vi "Dimostatore.vi"() -> ()   [LabVIEW 2019]
uses:
  ByteGSAPIBase/ByteGSAPIBase.lvclass
  ByteGSAPIBase/FetchCalibration/Converted_Slug_Cluster.ctl
  ByteGSAPIBase/CalibrationMeasurements/BodyCalibrazioneMisure.ctl
  6d3d0a70-a223-4ddd-b0d3-7207305fe689.vi
  85eea304-0067-4311-882a-d02f57de18c2.vi
panel:
  out "Valore misurato":string
  out "Valore di riferimento":string
  in  "Start":bool
  in  "Send":bool
  out "Infobox":string
  out "Strumenti da calibrare":i32(listbox)
  in  "Exit":bool=TRUE
  in  "Calibrate":bool
  in  "error out":errorcluster
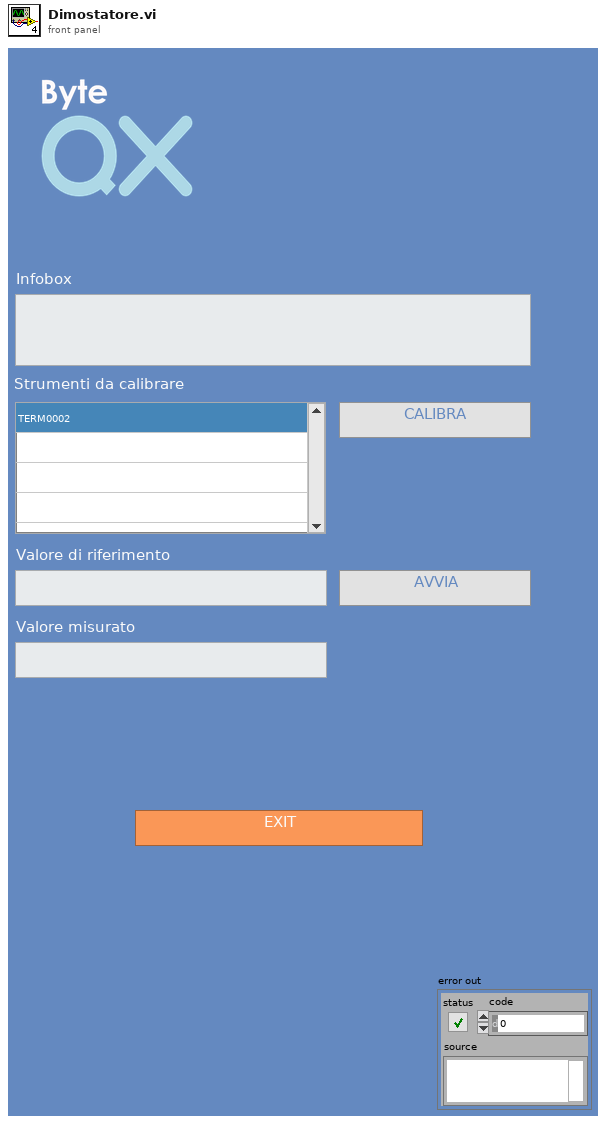
[diagram p1: front panel]
types:
  T1 = cluster{"nome":string, cluster{"Measurement_Id":i32, "Passed?":bool}[]}[]
  T2 = typedef "ByteGSWebAPI.lvlib/ByteGSAPIBase.lvclass/BodyCalibrazioneMisure.ctl" = cluster{"controls":cluster{"id":u16, "descrizione":string, "numero_misure_necessarie":u16, "riferimento_obiettivo":dbl, "mpe_max":dbl, "mpe_min":dbl, "deviazione_standard":dbl, "incertezza":dbl, "numero_misure_effettuate":u32, "temperatura_c":dbl, "umidita":dbl, "strumento_riferimento":cluster{"id":u16, "nome":string}[]}[]}
  T3 = typedef "ByteGSWebAPI.lvlib/ByteGSAPIBase.lvclass/Converted_Slug_Cluster.ctl" = cluster{"id":u32, "instrument":string, "name":string, "date":timestamp}
  T4 = cluster{"ByteGSAPIBase in":refnum<class "ByteGSAPIBase.lvclass">, "Expired_Instruments":T3[], "Calibrations":T2, "Strumenti_calibrati":cluster{"nome":string, cluster{"Measurement_Id":i32, "Passed?":bool}[]}[], "Instr_index":i32, "Calib_index":i32, "Instruments_Slug":string[], "ID_failed":u32, "Measure_Index":u32}
  T5 = cluster{"id":u16, "descrizione":string, "numero_misure_necessarie":u16, "riferimento_obiettivo":dbl, "mpe_max":dbl, "mpe_min":dbl, "deviazione_standard":dbl, "incertezza":dbl, "numero_misure_effettuate":u32, "temperatura_c":dbl, "umidita":dbl, "strumento_riferimento":cluster{"id":u16, "nome":string}[]}[]
  T6 = cluster{"id":u16, "descrizione":string, "numero_misure_necessarie":u16, "riferimento_obiettivo":dbl, "mpe_max":dbl, "mpe_min":dbl, "deviazione_standard":dbl, "incertezza":dbl, "numero_misure_effettuate":u32, "temperatura_c":dbl, "umidita":dbl, "strumento_riferimento":cluster{"id":u16, "nome":string}[]}
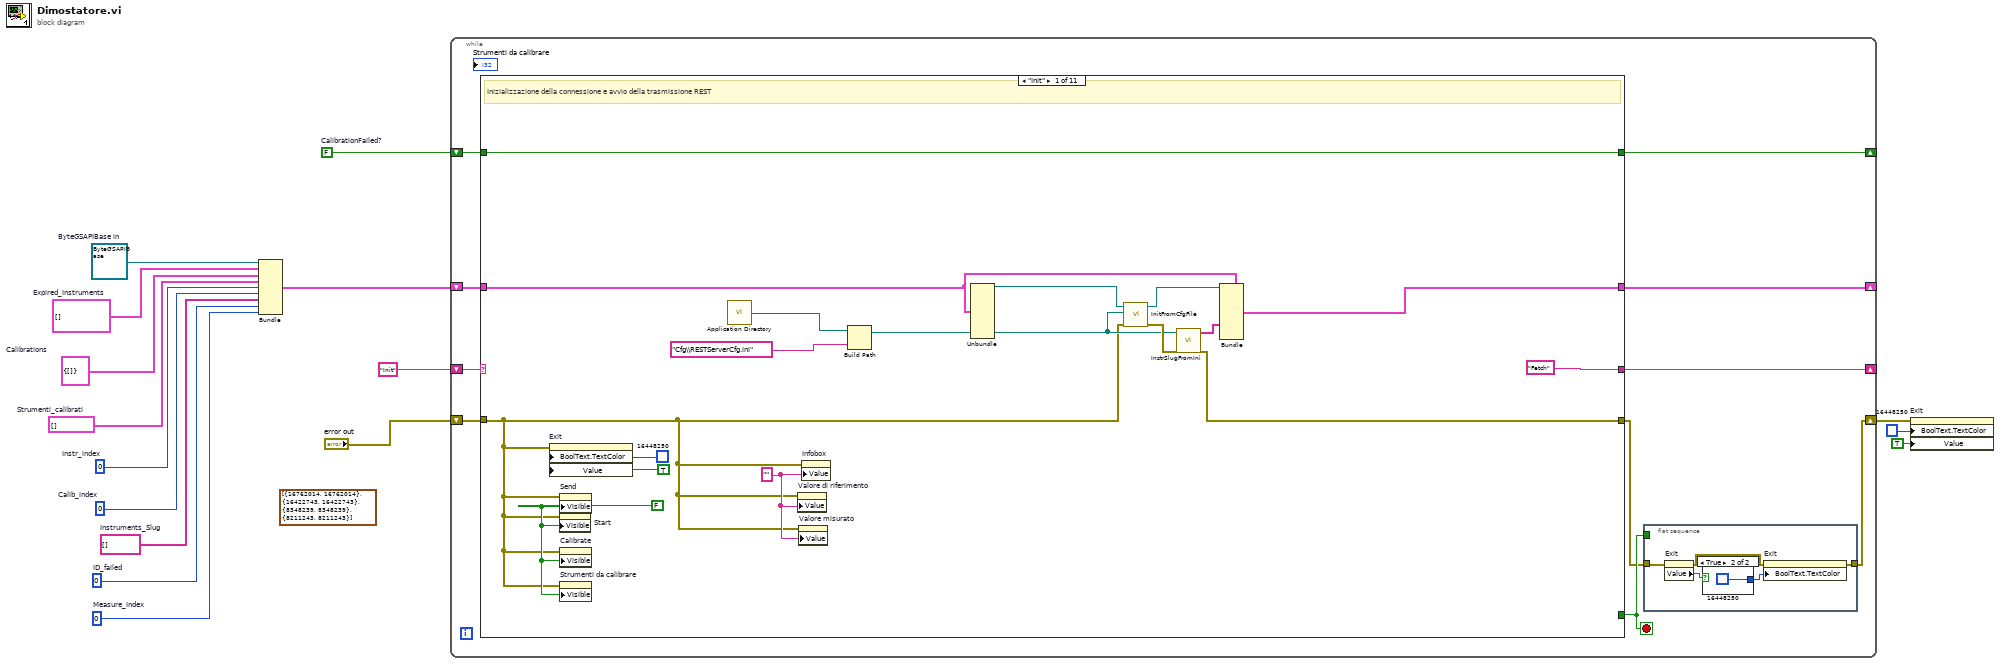
[diagram p0: block diagram]
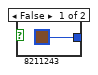
[diagram p2: hidden frame]
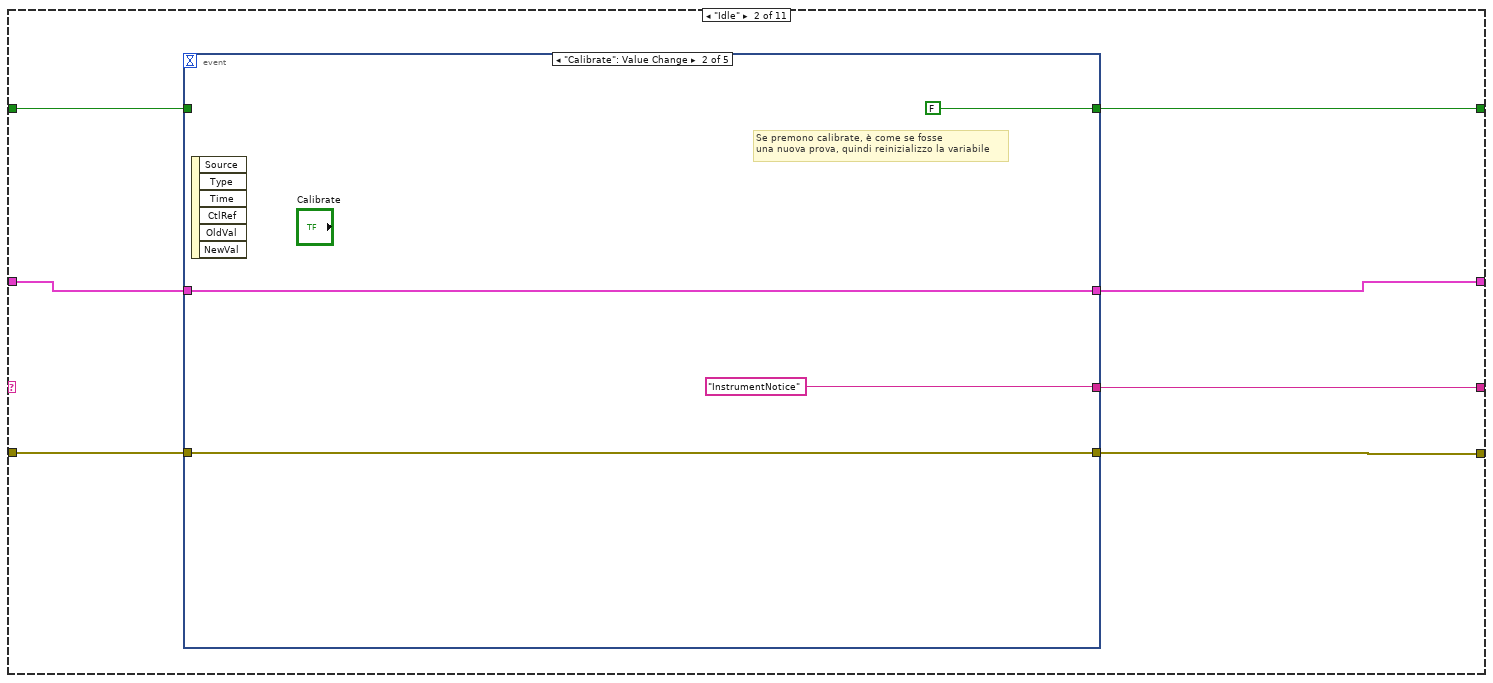
[diagram p3: hidden frame]
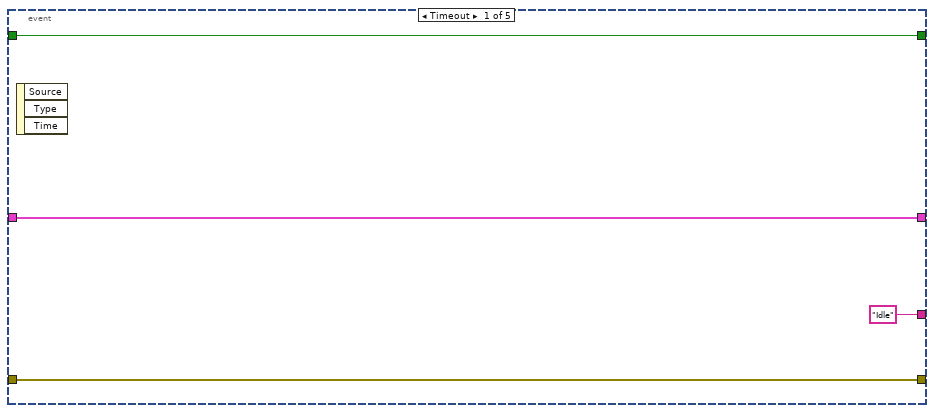
[diagram p4: hidden frame]
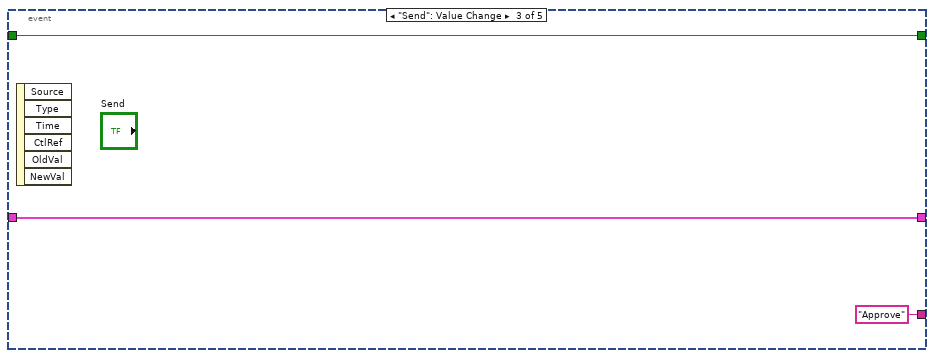
[diagram p5: hidden frame]
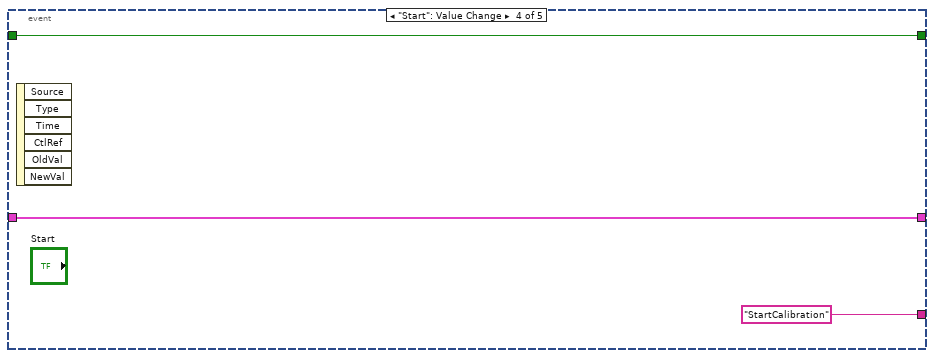
[diagram p6: hidden frame]
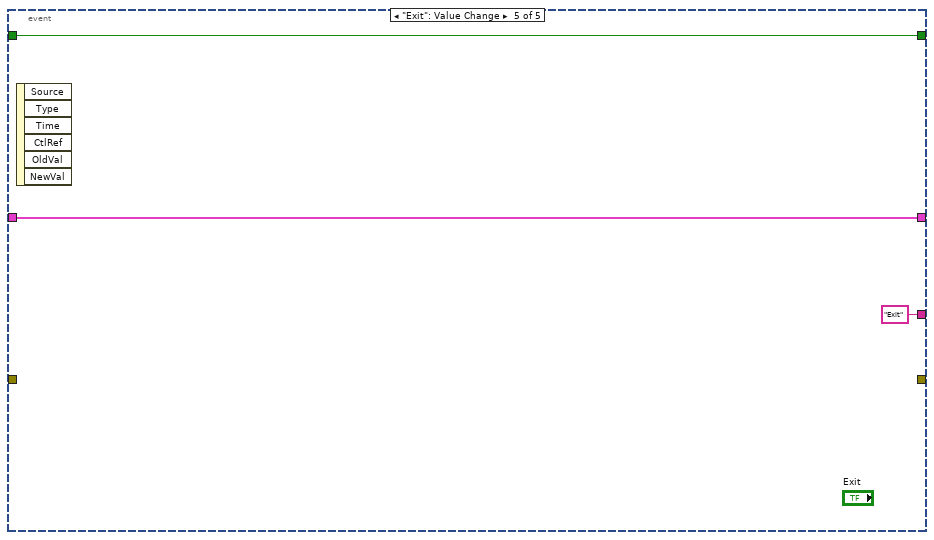
[diagram p7: hidden frame]
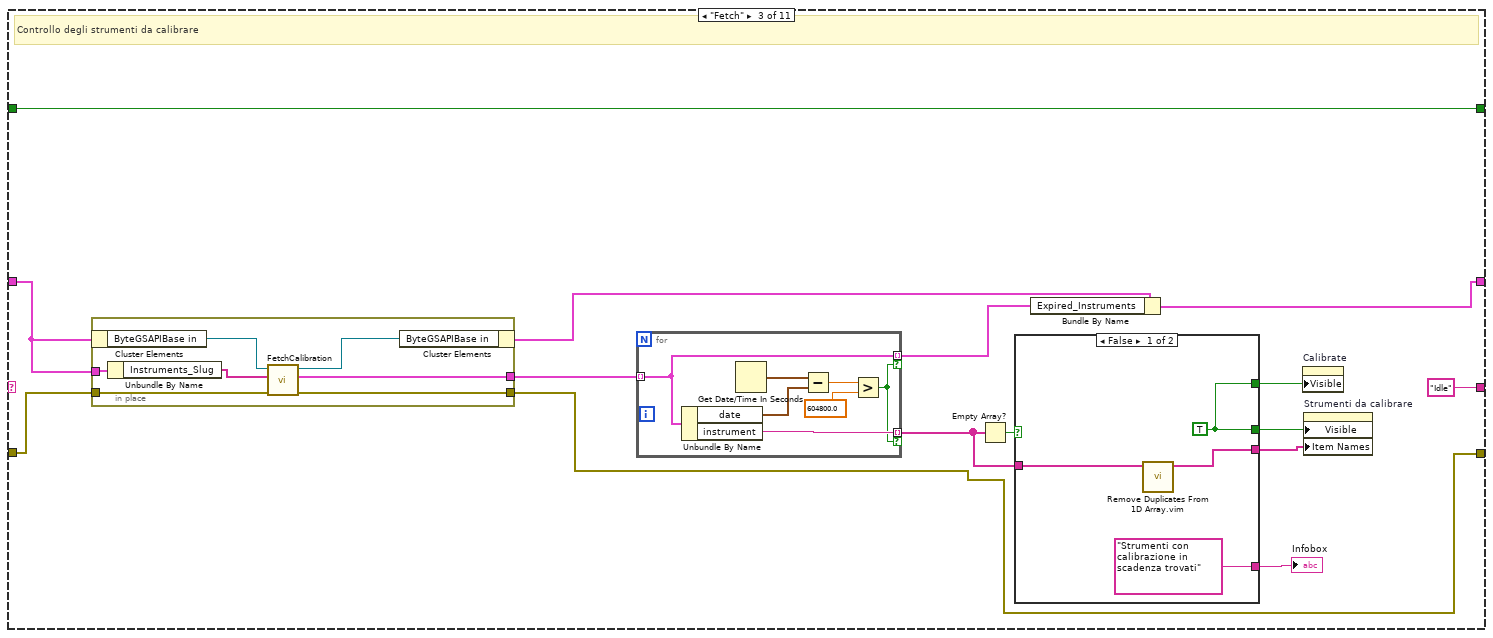
[diagram p8: hidden frame]
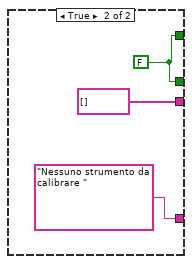
[diagram p9: hidden frame]
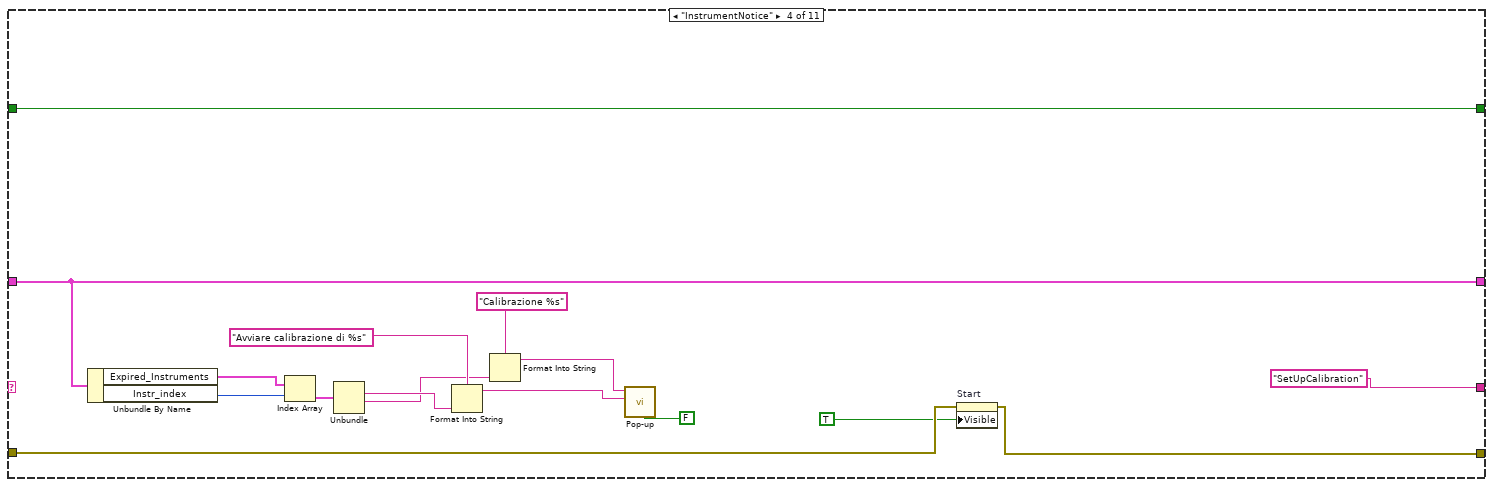
[diagram p10: hidden frame]
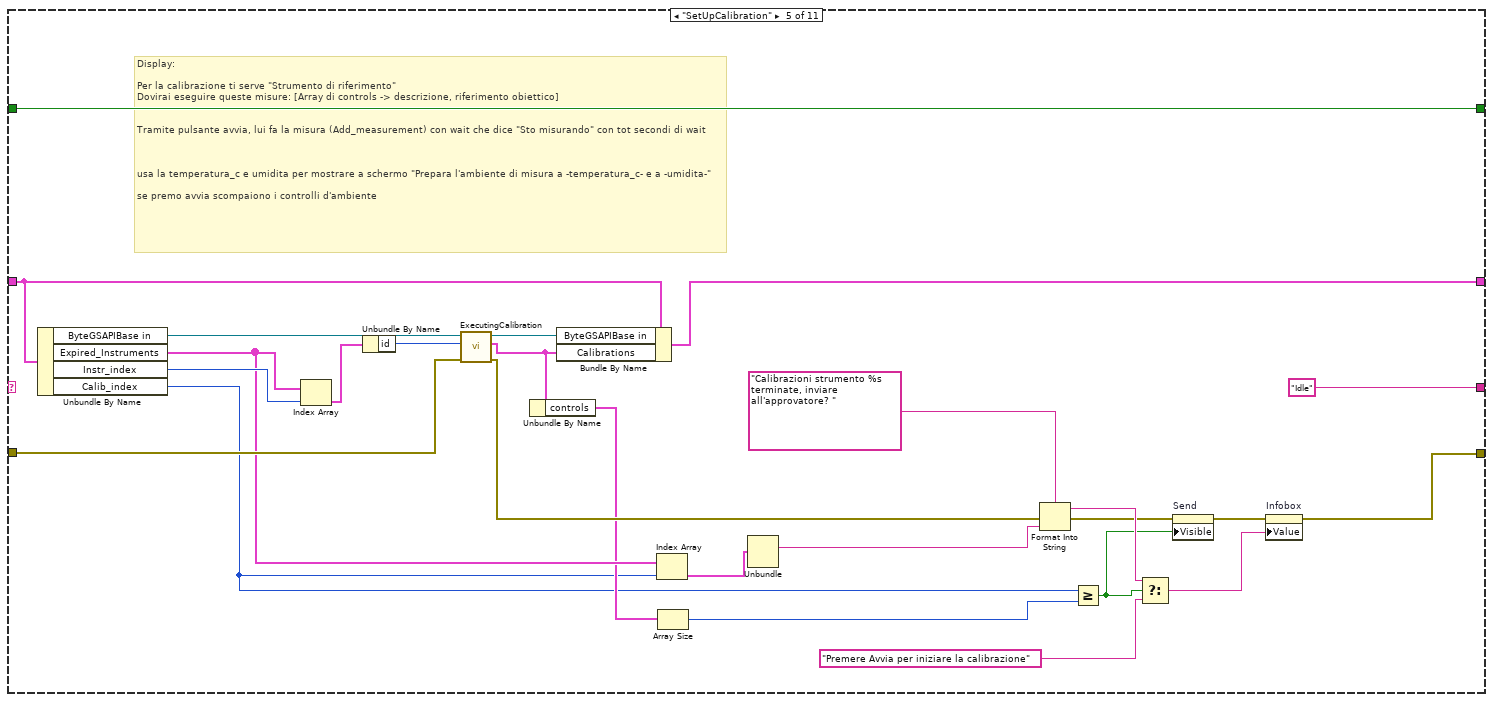
[diagram p11: hidden frame]
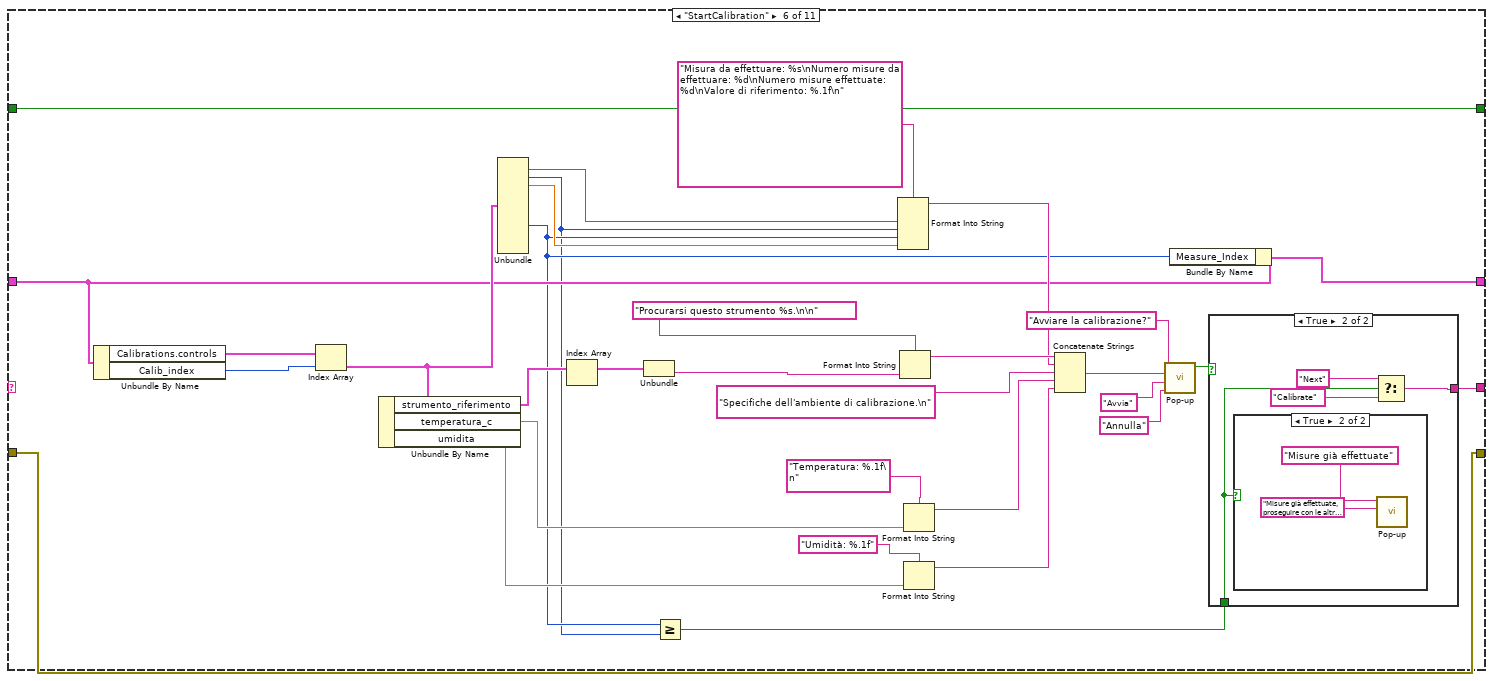
[diagram p12: hidden frame]
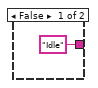
[diagram p13: hidden frame]
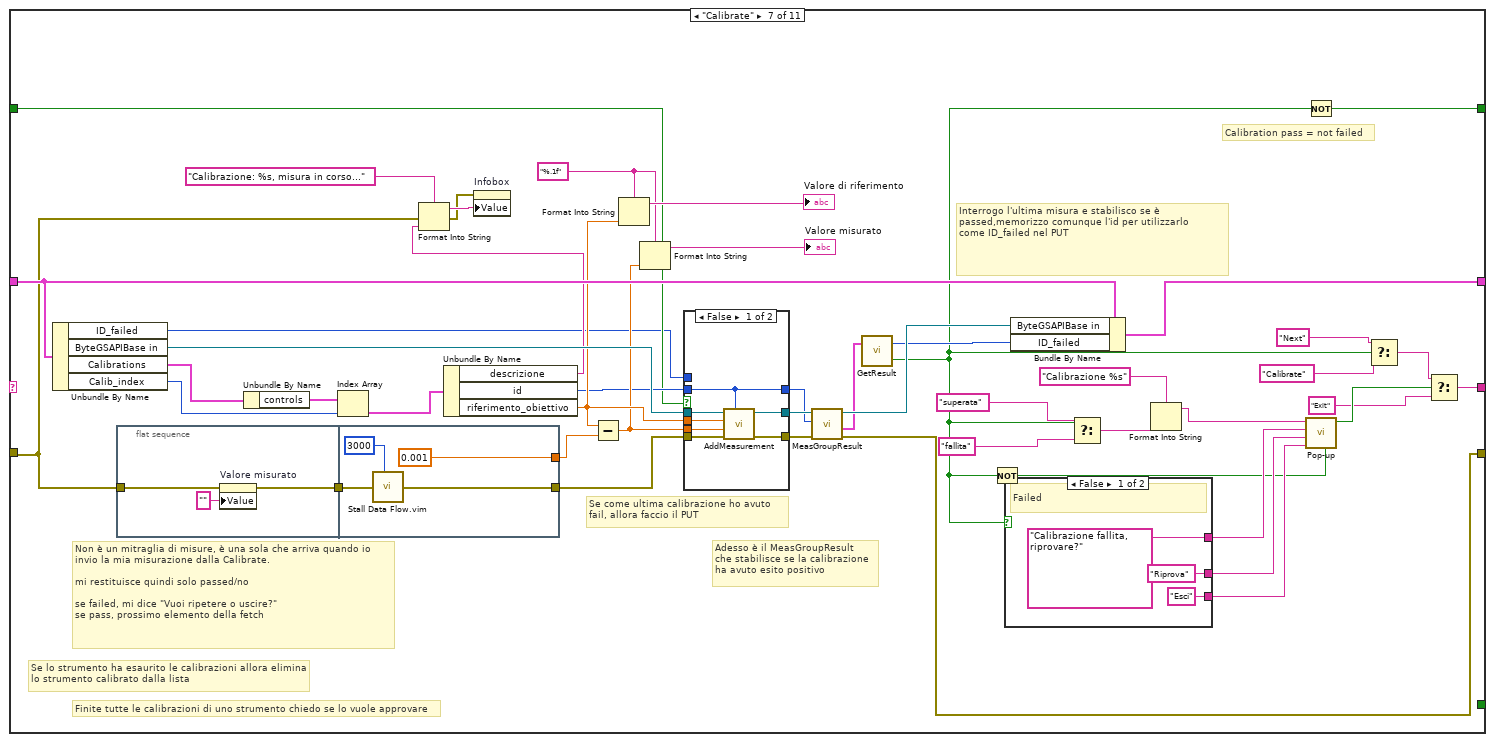
[diagram p15: hidden frame]
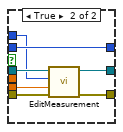
[diagram p16: hidden frame]
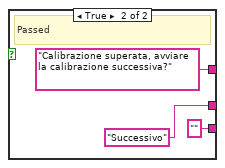
[diagram p17: hidden frame]
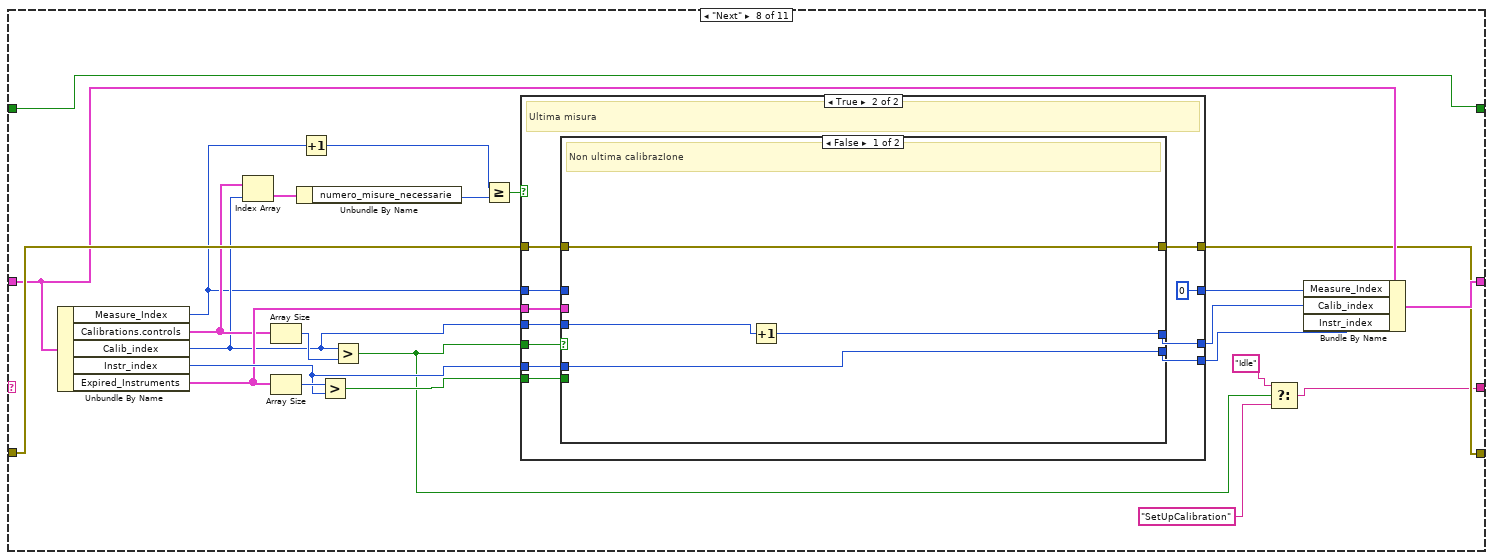
[diagram p18: hidden frame]
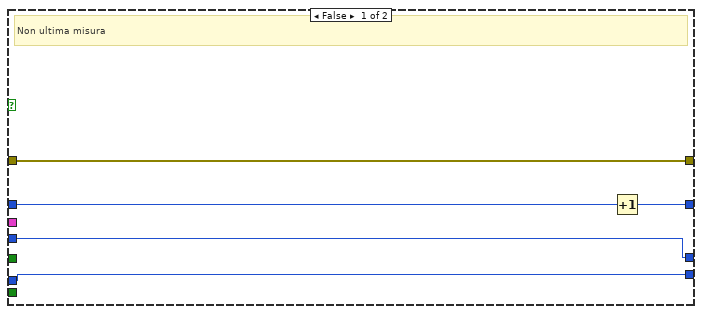
[diagram p19: hidden frame]
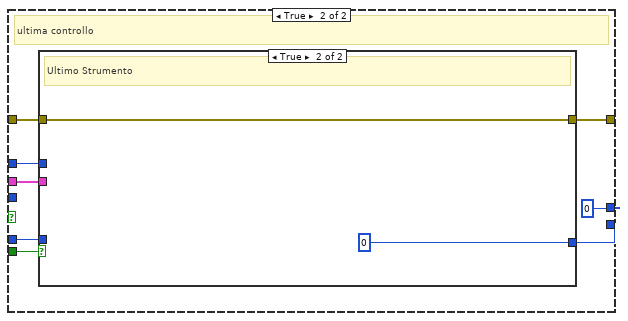
[diagram p20: hidden frame]
diagram:
  w1 = u32 0  # Measure_Index
  w2 = u32 0  # ID_failed
  w3 = FALSE  # CalibrationFailed?
  w4 = string[] []  # Instruments_Slug
  w8 = 0  # Calib_index
  w9 = 0  # Instr_index
  w10 = T1 []  # Strumenti_calibrati
  w11 = T2 {"controls"=[]}  # Calibrations
  (unwired) cluster{u32, u32}[] [{16762014, 16762014}, {16422743, 16422743}, {8348239, 8348239}, {8211243, 8211243}] ("Colors [4]")
  w12 = T3[] []  # Expired_Instruments
  w15 = refnum<class "ByteGSAPIBase.lvclass"> refnum  # ByteGSAPIBase in
  n1 = Bundle("ByteGSAPIBase in"=w15, "Expired_Instruments"=w12, "Calibrations"=w11, "Strumenti_calibrati"=w10, "Instr_index"=w9, "Calib_index"=w8, "Instruments_Slug"=w4, "ID_failed"=w2, "Measure_Index"=w1) -> (w14:T4)  [unwired: 1 in]
  n2 = while {
    shift-right: [w23] -> _
    shift-left: w14 -> [w25]
    shift-right: [w19] -> w7
    shift-left: "error out" -> [w24]
    shift-right: [w22] -> _
    shift-left: "Init" -> [w26]
    shift-right: [w17] -> _
    shift-left: w3 -> [w18]
    stop <- w21 stop-if-true
    n3 = case shown="\"Init\"" w26 {
      tunnel: w25 -> [w50 w54 w76 w126 w152 w157 w238 w282 w339 w352 w356]
      tunnel: w24 -> [w36 w56 w89 w114 w148 w176 w207 w283 w338 w353 w357]
      tunnel: [w39 w57 w77 w113 w144 w176 w203 w281 w324 w353 w357] -> w20
      tunnel: [w49 w55 w78 w126 w150 w156 w208 w288 w337 w352 w356] -> w23
      tunnel: [_ _ _ _ _ _ _ _ _ TRUE _] -> w21
      tunnel: ["Fetch" w53 "Idle" ("t") "SetUpCalibration" ("t") "Idle" ("t") w170 w214 w276 w331 "" ("t") "Exit" ("t")] -> w22
      tunnel: w18 -> [w35 w52 w75 w111 w130 w164 w198 w274 w323 w349 w354]
      tunnel: [w35 w51 w75 w111 w130 w164 w197 w274 w323 w349 w354] -> w17
      frame "Init" {
        w43 = "" ("Infobox")
        w42 = FALSE
        # "Inizializzazione della connessione e avvio della trasmissione REST"
        n4 = property on="Exit" class="Bool (strict)"(error in=w36, "BoolText.TextColor"=u32 16448250, "Value"=TRUE ("Exit")) -> ()  [unwired: 1 in, 2 out]
        n5 = property on="Start" class="Bool"(error in=w36, "Visible"=w42) -> ()  [unwired: 1 in, 2 out]
        n6 = property on="Send" class="Bool"(error in=w36, "Visible"=w42) -> ()  [unwired: 1 in, 2 out]
        n7 = property on="Calibrate" class="Bool"(error in=w36, "Visible"=w42) -> ()  [unwired: 1 in, 2 out]
        n8 = property on="Strumenti da calibrare" class="LstBox (strict)"(error in=w36, "Visible"=w42) -> ()  [unwired: 1 in, 2 out]
        n9 = call <vilib>:"Application Directory.vi"() -> ("Application Directory"=w34:path)
        n10 = property on="Valore di riferimento" class="Str"(error in=w36, "Value"=w43) -> ()  [unwired: 1 in, 2 out]
        n11 = property on="Valore misurato" class="Str"(error in=w36, "Value"=w43) -> ()  [unwired: 1 in, 2 out]
        n12 = property on="Infobox" class="Str"(error in=w36, "Value"=w43) -> ()  [unwired: 1 in, 2 out]
        n13 = Build Path(base path=w34, name or relative path="Cfg\\RESTServerCfg.ini") -> (appended path=w38:path)
        n14 = Unbundle(w50) -> ("ByteGSAPIBase in"=w45:refnum<class "ByteGSAPIBase.lvclass">)  [unwired: 8 out]
        n15 = call-dynamic "InitFromCfgFile.vi"("error in (no error)"=w36, "configuration file path"=w38, "ByteGSAPIBase in"=w45) -> ("error out"=w40:errorcluster, "ByteGSAPIBase out"=w44:refnum<class "ByteGSAPIBase.lvclass">)  [unwired: 7 in]
        n16 = call "InstrSlugFromIni.vi"("error in (no error)"=w40, "configuration file path"=w38) -> ("error out"=w39:errorcluster, "Array"=w37:string[])  [unwired: 8 in]
        n17 = Bundle(cluster=w50, "ByteGSAPIBase in"=w44, "Instruments_Slug"=w37) -> (w49:T4)  [unwired: 7 in]
      }
      frame "Idle" {
        n18 = event shown="[1] \"Calibrate\": Value Change" {
          selector: _ -> [_ _ _ _ _]
          dyn-events: _ -> [_ _ _ _ _]
          timeout: _ -> [_ _ _ _ _]
          tunnel: [w61 w63 _ _ _] -> w57
          tunnel: w56 -> [w61 w63 _ _ _]
          tunnel: [w60 w65 w68 w71 w74] -> w55
          tunnel: w54 -> [w60 w65 w68 w71 w74]
          tunnel: ["Idle" ("t") "InstrumentNotice" "Approve" ("t") "StartCalibration" ("t") "Exit" ("t")] -> w53
          tunnel: w52 -> [w58 _ w66 w69 w72]
          tunnel: [w58 FALSE ("CalibrationFailed?") w66 w69 w72] -> w51
          event Timeout {
            n19 = event-data() -> ()  [unwired: 1 in, 3 out]
          }
          event "Calibrate": Value Change {
            # "Se premono calibrate, è come se fosse\nuna nuova prova, quindi reinizializzo la variabile"
            n20 = event-data() -> ()  [unwired: 1 in, 6 out]
          }
          event "Send": Value Change {
            n21 = event-data() -> ()  [unwired: 1 in, 6 out]
          }
          event "Start": Value Change {
            n22 = event-data() -> ()  [unwired: 1 in, 6 out]
          }
          event "Exit": Value Change {
            n23 = event-data() -> ()  [unwired: 1 in, 6 out]
          }
        }
      }
      frame "Fetch" {
        # "Controllo degli strumenti da calibrare"
        n24 = in-place {
          in-place-border: w89 -> [w95]
          in-place-border: [w94] -> w77
          in-place-border: [w93] -> w81
          in-place-border: w76 -> [w91]
          n25 = in-place-cluster #1(w76) -> ("ByteGSAPIBase in"=w92:refnum<class "ByteGSAPIBase.lvclass">)
          n26 = Unbundle By Name(w91) -> ("Instruments_Slug"=w90:string[])
          n27 = call-dynamic "FetchCalibration.vi"("error in (no error)"=w95, "instruments"=w90, "ByteGSAPIBase in"=w92) -> ("error out"=w94:errorcluster, "instruments"=w93:T3[], "ByteGSAPIBase out"=w96:refnum<class "ByteGSAPIBase.lvclass">)  [unwired: 6 in]
          n28 = in-place-cluster #1("ByteGSAPIBase in"=w96) -> (w88:T4)
        }
        n29 = for {
          tunnel: w81 -> [w99] mode=indexing
          tunnel: [w99] -> w80 mode=indexing if=w97
          tunnel: [w98] -> w86 mode=indexing if=w97
          n30 = Unbundle By Name(w99) -> ("date"=w100:timestamp, "instrument"=w98:string)
          n31 = Get Date/Time In Seconds() -> (seconds since 1Jan1904=w102:timestamp)
          n32 = Subtract(x=w102, y=w100) -> (x-y=w103:dbl)
          n33 = Greater?(x=w103, y=604800.0) -> (0:w97:bool)
        }
        n34 = Empty Array?(array=w86) -> (empty?=w87:bool)
        n35 = case shown="False" w87 {
          tunnel: w86 -> [w106 _]
          tunnel: [w104 w108] -> w85
          tunnel: ["Strumenti con calibrazione in scadenza trovati" ("Infobox") "Nessuno strumento da calibrare " ("Infobox")] -> w84
          tunnel: [w105 string[] []] -> w83
          tunnel: [w104 w108] -> w79
          frame False {
            w104 = TRUE ("Visible")
            n36 = call "Remove Duplicates From 1D Array.vim"("array"=w106) -> ("array with duplicates removed"=w105:string[])  [unwired: 10 in]
          }
          frame True {
            w108 = FALSE ("Visible")
          }
        }
        "Infobox" <- w84
        n37 = Bundle By Name(cluster=w88, "Expired_Instruments"=w80) -> (w78:T4)
        n38 = property on="Calibrate" class="Bool"("Visible"=w79) -> ()  [unwired: 2 in, 2 out]
        n39 = property on="Strumenti da calibrare" class="LstBox (strict)"("Visible"=w85, "Item Names"=w83) -> ()  [unwired: 2 in, 2 out]
      }
      frame "InstrumentNotice" {
        n40 = Unbundle By Name(w126) -> ("Expired_Instruments"=w125:T3[], "Instr_index"=w124:i32)
        n41 = Index Array(array=w125, index=w124) -> (element=w123:T3)
        n42 = Unbundle(w123) -> ("instrument"=w121:string, "name"=w119:string)  [unwired: 2 out]
        n43 = Format Into String(format string="Avviare calibrazione di %s" ("Title"), w121) -> (resulting string=w120:string)  [unwired: 2 in, 1 out]
        n44 = Format Into String(format string="Calibrazione %s", w119) -> (resulting string=w117:string)  [unwired: 2 in, 1 out]
        n45 = call "Pop-up.vi"("Two_btn"=FALSE, "Text"=w120, "Title"=w117) -> ()  [unwired: 8 in, 1 out]
        n46 = property on="Start" class="Bool"(error in=w114, "Visible"=TRUE) -> (error out=w113:errorcluster)  [unwired: 1 in, 1 out]
      }
      frame "SetUpCalibration" {
        # "Display: \n\nPer la calibrazione ti serve \"Strumento di riferimento\"\nDovirai eseguire queste misure: [Array di controls -> descrizione, riferimento obiettico] \n\n\nTramite pulsante avvia, lui fa la misura (Add_measurement) con wait che dice \"Sto misurando\" con tot secondi di wait\n\n\n\nusa la temperatura_c e umidita per mostrare a schermo \"Prepara l'ambiente di misura a -temperatura_c- e a -umidita-\"\n\nse premo avvia scompaiono i controlli d'ambiente"
        n47 = Unbundle By Name(w152) -> ("ByteGSAPIBase in"=w151:refnum<class "ByteGSAPIBase.lvclass">, "Expired_Instruments"=w140:T3[], "Instr_index"=w145:i32, "Calib_index"=w128:i32)
        n48 = Index Array(array=w140, index=w145) -> (element=w146:T3)
        n49 = Unbundle By Name(w146) -> ("id"=w127:u32)
        n50 = call-dynamic "ExecutingCalibration.vi"("error in (no error)"=w148, "calibration_id"=w127, "ByteGSAPIBase in"=w151) -> ("error out"=w134:errorcluster, "calibration data"=w129:T2, "ByteGSAPIBase out"=w149:refnum<class "ByteGSAPIBase.lvclass">)  [unwired: 6 in]
        n51 = Unbundle By Name(w129) -> ("controls"=w131:T5)
        n52 = Bundle By Name(cluster=w152, "ByteGSAPIBase in"=w149, "Calibrations"=w129) -> (w150:T4)
        n53 = Index Array(array=w140, index=w128) -> (element=w141:T3)
        n54 = Array Size(array=w131) -> (size(s)=w138:i32)
        n55 = Unbundle(w141) -> ("instrument"=w139:string)  [unwired: 3 out]
        n56 = Format Into String(format string="Calibrazioni strumento %s terminate, inviare all'approvatore? ", error in=w134, w139) -> (resulting string=w143:string, error out=w133:errorcluster)  [unwired: 1 in]
        n57 = Greater Or Equal?(x=w128, y=w138) -> (x >= y?=w135:bool)
        n58 = Select(t=w143, s=w135, f="Premere Avvia per iniziare la calibrazione" ("Infobox")) -> (s? t:f=w136:string)
        n59 = property on="Send" class="Bool"(error in=w133, "Visible"=w135) -> (error out=w132:errorcluster)  [unwired: 1 in, 1 out]
        n60 = property on="Infobox" class="Str"(error in=w132, "Value"=w136) -> (error out=w144:errorcluster)  [unwired: 1 in, 1 out]
      }
      frame "StartCalibration" {
        n61 = Unbundle By Name(w157) -> ("Calibrations.controls"=w168:T5, "Calib_index"=w169:i32)
        n62 = Index Array(array=w168, index=w169) -> (element=w163:T6)
        n63 = Unbundle By Name(w163) -> ("strumento_riferimento"=w160:cluster{"id":u16, "nome":string}[], "temperatura_c"=w162:dbl, "umidita"=w161:dbl)
        n64 = Unbundle(w163) -> ("descrizione"=w166:string, "numero_misure_necessarie"=w154:u16, "riferimento_obiettivo"=w158:dbl, "numero_misure_effettuate"=w155:u32)  [unwired: 8 out]
        n65 = Index Array(array=w160) -> (element=w159:cluster{"id":u16, "nome":string})  [unwired: 1 in]
        n66 = Unbundle(w159) -> ("nome"=w178:string)  [unwired: 1 out]
        n67 = Greater Or Equal?(x=w155, y=w154) -> (x >= y?=w153:bool)
        n68 = Format Into String(format string="Misura da effettuare: %s\nNumero misure da effettuare: %d\nNumero misure effettuate: %d\nValore di riferimento: %.1f\n", w166, w154, w155, w158) -> (resulting string=w167:string)  [unwired: 2 in, 1 out]
        n69 = Format Into String(format string="Procurarsi questo strumento %s.\n\n", w178) -> (resulting string=w184:string)  [unwired: 2 in, 1 out]
        n70 = Format Into String(format string="Temperatura: %.1f\n", w162) -> (resulting string=w175:string)  [unwired: 2 in, 1 out]
        n71 = Format Into String(format string="Umidità: %.1f", w161) -> (resulting string=w173:string)  [unwired: 2 in, 1 out]
        n72 = Concatenate Strings(w184, w167, "Specifiche dell'ambiente di calibrazione.\n" ("string"), w175, w173) -> (w179:string)
        n73 = call "Pop-up.vi"("CancelText"="Annulla", "OkText"="Avvia", "Text"=w179, "Title"="Avviare la calibrazione?") -> ("Btn-OK Out"=w171:bool)  [unwired: 7 in]
        n74 = Bundle By Name(cluster=w157, "Measure_Index"=w155) -> (w156:T4)
        n75 = case shown="True" w171 {
          tunnel: ["Idle" w187] -> w170
          tunnel: w153 -> [_ w186]
          frame False {
          }
          frame True {
            n76 = case shown="True" w186 {
              frame False {
              }
              frame True {
                n77 = call "Pop-up.vi"("Text"="Misure già effettuate, proseguire con le altre tarature" ("Title"), "Title"="Misure già effettuate") -> ()  [unwired: 9 in, 1 out]
              }
            }
            n78 = Select(t="Next", s=w186, f="Calibrate") -> (s? t:f=w187:string)
          }
        }
      }
      frame "Calibrate" {
        w227 = "%.1f" ("format string")
        # "Interrogo l'ultima misura e stabilisco se è passed,memorizzo comunque l'id per utilizzarlo\ncome ID_failed nel PUT"
        # "Calibration pass = not failed"
        # "Se come ultima calibrazione ho avuto\nfail, allora faccio il PUT"
        # "Adesso è il MeasGroupResult\nche stabilisce se la calibrazione\nha avuto esito positivo"
        # "Finite tutte le calibrazioni di uno strumento chiedo se lo vuole approvare"
        # "Se lo strumento ha esaurito le calibrazioni allora elimina\nlo strumento calibrato dalla lista"
        # "Non è un mitraglia di misure, è una sola che arriva quando io\ninvio la mia misurazione dalla Calibrate.\n\nmi restituisce quindi solo passed/no \n\nse failed, mi dice \"Vuoi ripetere o uscire?\"\nse pass, prossimo elemento della fetch"
        n79 = Unbundle By Name(w238) -> ("ID_failed"=w192:u32, "ByteGSAPIBase in"=w237:refnum<class "ByteGSAPIBase.lvclass">, "Calibrations"=w236:T2, "Calib_index"=w230:i32)
        n80 = flat-sequence {
          tunnel: w207 -> [w254]
          tunnel: [w255] -> w205
          tunnel: [0.001 ("number: 0 to 1")] -> w225
          tunnel: [w257] -> w206
          tunnel: w205 -> [w258]
          frame #0 {
            n81 = property on="Valore misurato" class="Str"(error in=w254, "Value"="" ("Valore misurato")) -> (error out=w255:errorcluster)  [unwired: 1 in, 1 out]
          }
          frame #1 {
            n82 = call "Stall Data Flow.vim"("value in"=w258, "milliseconds to wait"=u32 3000) -> ("value out"=w257:errorcluster)  [unwired: 1 out]
          }
        }
        n83 = Unbundle By Name(w236) -> ("controls"=w231:T5)
        n84 = Index Array(array=w231, index=w230) -> (element=w232:T6)
        n85 = Unbundle By Name(w232) -> ("descrizione"=w196:string, "id"=w202:u16, "riferimento_obiettivo"=w229:dbl)
        n86 = Format Into String(format string="Calibrazione: %s, misura in corso...", error in=w207, w196) -> (resulting string=w235:string, error out=w234:errorcluster)  [unwired: 1 in]
        n87 = property on="Infobox" class="Str"(error in=w234, "Value"=w235) -> ()  [unwired: 1 in, 2 out]
        n88 = Subtract(x=w229, y=w225) -> (x-y=w209:dbl)
        n89 = Format Into String(format string=w227, w229) -> (resulting string=→"Valore di riferimento":string)  [unwired: 2 in, 1 out]
        n90 = Format Into String(format string=w227, w209) -> (resulting string=→"Valore misurato":string)  [unwired: 2 in, 1 out]
        n91 = case shown="False" w198 {
          tunnel: w237 -> [w245 w252]
          tunnel: w229 -> [w244 _]
          tunnel: w209 -> [w243 w250]
          tunnel: w206 -> [w242 w251]
          tunnel: [w241 w248] -> w204
          tunnel: w202 -> [w239 w247]
          tunnel: [w240 w249] -> w201
          tunnel: [w239 w247] -> w199
          tunnel: w192 -> [_ w246]
          frame False {
            n92 = call-dynamic "AddMeasurement.vi"("measurement-group-id"=w239, "error in (no error)"=w242, "instrument measure"=w243, "reference measure"=w244, "ByteGSAPIBase in"=w245) -> ("error out"=w241:errorcluster, "ByteGSAPIBase out"=w240:refnum<class "ByteGSAPIBase.lvclass">)  [unwired: 4 in, 1 out]
          }
          frame True {
            n93 = call-dynamic "EditMeasurement.vi"("error in (no error)"=w251, "instrument measure"=w250, "measurement-id"=w246, "ByteGSAPIBase in"=w252) -> ("error out"=w248:errorcluster, "ByteGSAPIBase out"=w249:refnum<class "ByteGSAPIBase.lvclass">)  [unwired: 5 in, 1 out]
          }
        }
        n94 = call-dynamic "MeasGroupResult.vi"("error in (no error)"=w204, "measurement_group_id"=w199, "ByteGSAPIBase in"=w201) -> ("error out"=w203:errorcluster, "measurements"=w195:cluster{"id":u32, "passed":bool}[], "ByteGSAPIBase out"=w200:refnum<class "ByteGSAPIBase.lvclass">)  [unwired: 5 in, 1 out]
        n95 = call "GetResult.vi"("measurements"=w195) -> ("passed"=w193:bool, "id"=w194:u32)  [unwired: 1 in]
        n96 = Not(x=w193) -> (.not. x?=w213:bool)
        n97 = case shown="False" w193 {
          tunnel: ["Riprova" "Successivo"] -> w219
          tunnel: ["Esci" ""] -> w218
          tunnel: ["Calibrazione fallita, riprovare?" ("Text") "Calibrazione superata, avviare la calibrazione successiva?" ("Text")] -> w217
          frame False {
            # "Failed"
          }
          frame True {
            # "Passed"
          }
        }
        n98 = Bundle By Name(cluster=w238, "ByteGSAPIBase in"=w200, "ID_failed"=w194) -> (w208:T4)
        n99 = Select(t="superata", s=w193, f="fallita") -> (s? t:f=w223:string)
        n100 = Format Into String(format string="Calibrazione %s", w223) -> (resulting string=w220:string)  [unwired: 2 in, 1 out]
        n101 = Not(x=w193) -> (.not. x?=w197:bool)
        n102 = call "Pop-up.vi"("Two_btn"=w213, "CancelText"=w218, "OkText"=w219, "Text"=w217, "Title"=w220) -> ("Btn-OK Out"=w216:bool)  [unwired: 6 in]
        n103 = Select(t="Next", s=w193, f="Calibrate") -> (s? t:f=w211:string)
        n104 = Select(t=w211, s=w216, f="Exit") -> (s? t:f=w214:string)
      }
      frame "Next" {
        n105 = Unbundle By Name(w282) -> ("Measure_Index"=w268:u32, "Calibrations.controls"=w273:T5, "Calib_index"=w272:i32, "Instr_index"=w284:i32, "Expired_Instruments"=w280:T3[])
        n106 = Index Array(array=w273, index=w272) -> (element=w271:T6)
        n107 = Array Size(array=w273) -> (size(s)=w289:i32)
        n108 = Array Size(array=w280) -> (size(s)=w286:i32)
        n109 = Unbundle By Name(w271) -> ("numero_misure_necessarie"=w270:u16)
        n110 = Increment(x=w268) -> (x+1=w266:u32)
        n111 = Greater?(x=w286, y=w284) -> (0:w279:bool)
        n112 = Greater?(x=w272, y=w289) -> (0:w275:bool)
        n113 = Greater Or Equal?(x=w266, y=w270) -> (x >= y?=w269:bool)
        n114 = case shown="True" w269 {
          tunnel: [w294 w305] -> w287
          tunnel: [w293 w304] -> w285
          tunnel: w272 -> [w294 w303]
          tunnel: w284 -> [w293 w302]
          tunnel: w283 -> [w290 w301]
          tunnel: [w290 w300] -> w281
          tunnel: w280 -> [_ w299]
          tunnel: w279 -> [_ w298]
          tunnel: w275 -> [_ w297]
          tunnel: w268 -> [w292 w295]
          tunnel: [w291 u32 0] -> w267
          frame False {
            # "Non ultima misura"
            n115 = Increment(x=w292) -> (x+1=w291:u32)
          }
          frame True {
            # "Ultima misura"
            n116 = case shown="False" w297 {
              tunnel: [w308 0 ("Calib_index")] -> w305
              tunnel: w303 -> [w309 _]
              tunnel: w302 -> [w307 w315]
              tunnel: w298 -> [_ w317]
              tunnel: [w307 w314] -> w304
              tunnel: w301 -> [w306 w313]
              tunnel: [w306 w312] -> w300
              tunnel: w299 -> [_ w311]
              tunnel: w295 -> [_ w310]
              frame False {
                # "Non ultima calibrazIone"
                n117 = Increment(x=w309) -> (x+1=w308:i32)
              }
              frame True {
                # "ultima controllo"
                n118 = case shown="True" w317 {
                  tunnel: w315 -> [w320 _]
                  tunnel: [w319 0] -> w314
                  tunnel: w313 -> [w318 w321]
                  tunnel: [w318 w321] -> w312
                  tunnel: w311 -> [_ _]
                  tunnel: w310 -> [_ _]
                  frame False {
                    n119 = Increment(x=w320) -> (x+1=w319:i32)
                  }
                  frame True {
                    # "Ultimo Strumento"
                  }
                }
              }
            }
          }
        }
        n120 = Select(t="Idle", s=w275, f="SetUpCalibration") -> (s? t:f=w276:string)
        n121 = Bundle By Name(cluster=w282, "Measure_Index"=w267, "Calib_index"=w287, "Instr_index"=w285) -> (w288:T4)
      }
      frame "Approve" {
        n122 = in-place {
          in-place-border: w339 -> [w346]
          in-place-border: w338 -> [w345]
          in-place-border: [w344] -> w325
          n123 = in-place-cluster #2(w339) -> ("ByteGSAPIBase in"=w348:refnum<class "ByteGSAPIBase.lvclass">)
          n124 = Unbundle By Name(w346) -> ("Expired_Instruments"=w343:T3[], "Instr_index"=w342:i32)
          n125 = Index Array(array=w343, index=w342) -> (element=w341:T3)
          n126 = Unbundle(w341) -> ("id"=w340:u32)  [unwired: 3 out]
          n127 = call-dynamic "RequestApproval.vi"("error in (no error)"=w345, "calibration-id"=w340, "ByteGSAPIBase in"=w348) -> ("error out"=w344:errorcluster, "ByteGSAPIBase out"=w347:refnum<class "ByteGSAPIBase.lvclass">)  [unwired: 6 in, 1 out]
          n128 = in-place-cluster #2("ByteGSAPIBase in"=w347) -> (w337:T4)
        }
        n129 = Unbundle(w337) -> ("Expired_Instruments"=w336:T3[], "Instr_index"=w334:i32)  [unwired: 7 out]
        n130 = Array Size(array=w336) -> (size(s)=w335:i32)
        n131 = Less Or Equal?(x=w335, y=w334) -> (x <= y?=w328:bool)
        n132 = Not(x=w328) -> (.not. x?=w327:bool)
        n133 = Select(t="InstrumentNotice", s=w328, f="Idle") -> (s? t:f=w331:string)
        n134 = Select(t="Tutte le calibrazioni terminate", s=w327, f="") -> (s? t:f=w326:string)
        n135 = property on="Infobox" class="Str"(error in=w325, "Value"=w326) -> (error out=w324:errorcluster)  [unwired: 1 in, 1 out]
      }
      frame "Exit" {
        # "Uscita"
      }
      frame Default {
        # "Qua non dovrebbe entrarci"
      }
    }
    n136 = flat-sequence {
      tunnel: w21 -> [_]
      tunnel: [w29] -> w19
      tunnel: w20 -> [w28]
      frame #0 {
        n137 = property on="Exit" class="Bool (strict)"(error in=w28) -> (error out=w27:errorcluster, "Value"=w30:bool)  [unwired: 1 in, 1 out]
        n138 = case shown="True" w30 {
          tunnel: [u32 8211243 u32 16448250 ("Boolean Text.Text Colors:Text Color")] -> w31
          frame False {
          }
          frame True {
          }
        }
        n139 = property on="Exit" class="Bool (strict)"(error in=w27, "BoolText.TextColor"=w31) -> (error out=w29:errorcluster)  [unwired: 1 in, 1 out]
      }
    }
  }
  n140 = property on="Exit" class="Bool (strict)"(error in=w7, "BoolText.TextColor"=u32 16448250 ("Boolean Text.Text Colors:Text Color"), "Value"=TRUE ("Exit")) -> ()  [unwired: 1 in, 2 out]
